vi "SynapseAPI-Create Subject.vi"(0 "URL":string="http://localhost:24414", 5 "subject":string, 7 "desc":string, 9 "icon":string="mouse", 11 "error in (no error)":errorcluster) -> (15 "error out":errorcluster)   [LabVIEW 2020]
uses:
  <vilib>/httpClient/PUTBuffer.vi
  <vilib>/httpClient/LabVIEWHTTPClient.lvlib
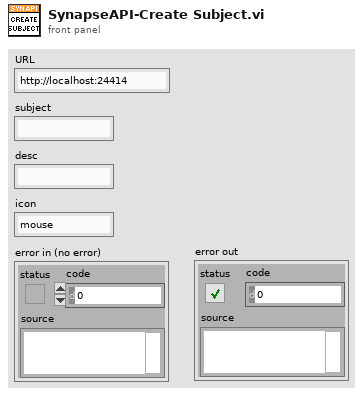
[diagram p1: front panel]
types:
  T1 = cluster{"subject":string, "desc":string, "icon":string}
  T2 = typedef "LabVIEWHTTPClient.lvlib/ClientHandle.ctl" = refnum<k1>
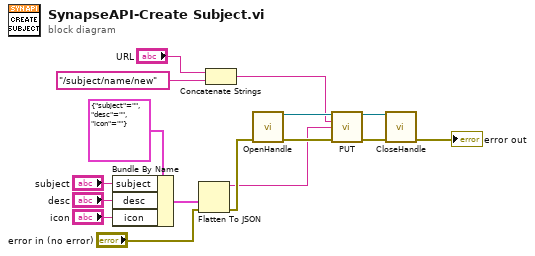
[diagram p0: block diagram]
diagram:
  n1 = Bundle By Name(cluster=T1 {"subject"="", "desc"="", "icon"=""} ("Cluster"), "subject"="subject", "desc"="desc", "icon"="icon") -> (w15:T1)
  n2 = Flatten To JSON(anything=w15, error in (no error)="error in (no error)") -> (JSON string=w6:string, 11:w7:errorcluster)  [unwired: 1 in]
  n3 = Concatenate Strings("URL", "/subject/name/new") -> (w8:string)
  n4 = call <vilib>:"OpenHandle.vi"("error in (no error)"=w7) -> ("client handle out"=w11:T2, "error out"=w10:errorcluster)  [unwired: 13 in]
  n5 = call-poly <vilib>:"PUT.vi"("client handle"=w11, "url"=w8, "buffer"=w6, "error in (no error)"=w10) -> ("client handle out"=w13:T2, "error out"=w14:errorcluster)  [unwired: 8 in, 2 out]
  n6 = call <vilib>:"CloseHandle.vi"("client handle"=w13, "error in (no error)"=w14) -> ("error out"=→"error out":errorcluster)  [unwired: 13 in]
